vi "ep_Peak Search in Window.vi"(6 "fr when 1 polepairs? (F)":bool, 8 "error in (no error)":errorcluster, 9 "frequency excluded":dbl[](array[numeric]), 10 "magnitude in window":dbl[](array[numeric]), 11 "frequency in window":dbl[](array[numeric])) -> (0 "error out":errorcluster, 2 "number of peaks":i32, 3 "peaks information":T1)   [LabVIEW 2014, in "NI_EP_Motor Monitoring.lvlib"]
uses:
  <vilib>/addons/Electrical Power/Motor Monitoring/NI_EP_Motor Monitoring.lvlib
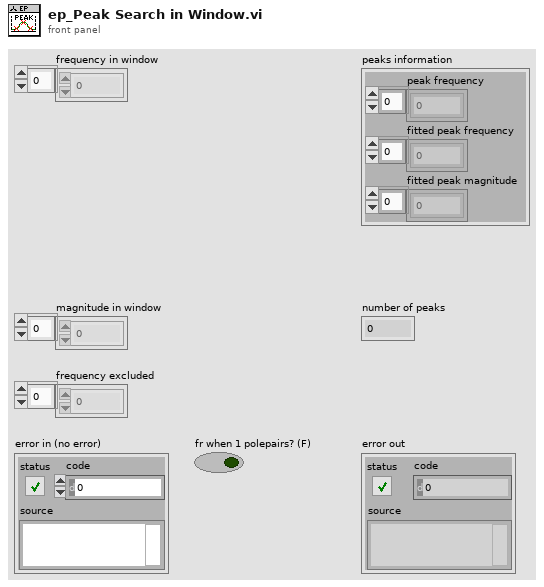
[diagram p1: front panel]
types:
  T1 = cluster{"peak frequency":dbl[], "fitted peak frequency":dbl[], "fitted peak magnitude":dbl[]}
  T2 = cluster{"original peak frequency":dbl[], "fitted peak frequency":dbl[], "fitted peak magnitude":dbl[]}
  T3 = cluster{"maximum frequency [Hz]":dbl, "slip error allowance":dbl, "minimum points for peak search":dbl, "accuracy of fs":dbl, "difference?":bool, " fs harmonics order":i32, "fs forbidden range":dbl, "p3:p1 valid significance ratio":dbl, "ratio for significance weighting":dbl, "significance weighting":dbl}
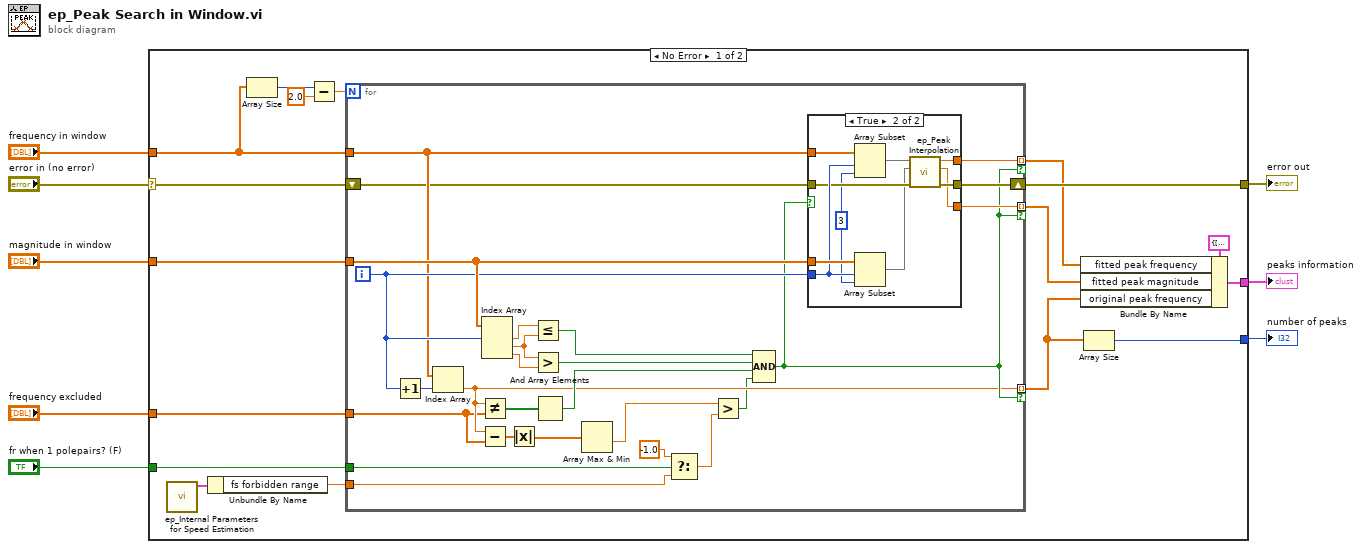
[diagram p0: block diagram]
diagram:
  n1 = case shown="No Error" "error in (no error)" {
    selector: "error in (no error)" -> [w9 w63]
    tunnel: "magnitude in window" -> [w14 _]
    tunnel: "frequency excluded" -> [w10 _]
    tunnel: "frequency in window" -> [w22 _]
    tunnel: [w21 w63] -> w4
    tunnel: [w20 _] -> w3
    tunnel: [w19 _] -> w2
    tunnel: "fr when 1 polepairs? (F)" -> [w13 _]
    frame No Error {
      n2 = call <vilib>:"ep_Internal Parameters for Speed Estimation.vi"() -> ("internal parameters for speed estimation"=w12:T3)  [unwired: 11 in]
      n3 = Unbundle By Name(w12) -> ("fs forbidden range"=w11:dbl)
      n4 = Array Size(array=w22) -> (size(s)=w24:i32)
      n5 = Subtract(x=w24, y=2.0) -> (x-y=w23:dbl)
      n6 = for {
        N: w23 -> [_]
        tunnel: w22 -> [w45]
        tunnel: w14 -> [w47]
        tunnel: w10 -> [w34]
        shift-right: [w44] -> w21
        shift-left: w9 -> [w43]
        tunnel: [w39] -> w18 mode=indexing if=w36
        tunnel: [w38] -> w17 mode=indexing if=w36
        tunnel: [w35] -> w15 mode=indexing if=w36
        tunnel: w13 -> [w27]
        tunnel: w11 -> [w26]
        i -> [w46]
        n7 = Increment(x=w46) -> (x+1=w49:i32)
        n8 = Index Array(array=w45, index=w49) -> (element=w35:dbl)
        n9 = Not Equal?(x=w35, y=w34) -> (x != y?=w48:bool[])
        n10 = Subtract(x=w35, y=w34) -> (x-y=w33:dbl[])
        n11 = Index Array(array=w47, index #1=w46) -> (element #1=w50:dbl, element #2=w37:dbl, element #3=w51:dbl)  [unwired: 2 in]
        n12 = Absolute Value(x=w33) -> (abs(x)=w32:dbl[])
        n13 = Less Or Equal?(x=w50, y=w37) -> (x <= y?=w42:bool)
        n14 = Greater?(x=w37, y=w51) -> (0:w41:bool)
        n15 = And Array Elements(Boolean array=w48) -> (logical AND=w40:bool)
        n16 = Array Max & Min(array=w32) -> (min value=w30:dbl)  [unwired: 3 out]
        n17 = Select(t=-1.0 ("x"), s=w27, f=w26) -> (s? t:f=w28:dbl)
        n18 = Greater?(x=w30, y=w28) -> (0:w31:bool)
        n19 = Compound Arithmetic op=AND(w42, w41, w40, w31) -> (w36:bool)
        n20 = case shown="True" w36 {
          tunnel: w47 -> [_ w62]
          tunnel: w46 -> [_ w61]
          tunnel: w45 -> [_ w60]
          tunnel: [w52 w58] -> w44
          tunnel: w43 -> [w52 w57]
          tunnel: [_ w55] -> w39
          tunnel: [_ w54] -> w38
          frame False {
          }
          frame True {
            w56 = 3 ("length")
            n21 = Array Subset(array=w60, index=w61, length=w56) -> (w59:dbl[])
            n22 = Array Subset(array=w62, index=w61, length=w56) -> (w53:dbl[])
            n23 = call <vilib>:"ep_Peak Interpolation.vi"("error in (no error)"=w57, "magnitude"=w53, "frequency [Hz]"=w59) -> ("error out"=w58:errorcluster, "fitted peak magnitude"=w54:dbl, "fitted peak frequency"=w55:dbl)  [unwired: 6 in]
          }
        }
      }
      n24 = Bundle By Name(cluster=T2 {"original peak frequency"=[], "fitted peak frequency"=[], "fitted peak magnitude"=[]} ("Cluster"), "fitted peak frequency"=w18, "fitted peak magnitude"=w17, "original peak frequency"=w15) -> (w20:T2)
      n25 = Array Size(array=w15) -> (size(s)=w19:i32)
    }
    frame Error {
    }
  }
  "error out" <- w4
  "peaks information" <- w3
  "number of peaks" <- w2
